vi "生成报告old.vi"() -> ()   [LabVIEW 2013]
uses:
  <vilib>/Utility/NIReport.llb/NI_report.lvclass
  <vilib>/Utility/NIReport.llb/Append Report Text (str wrap).vi
  <vilib>/Utility/NIReport.llb/Append Image to Report (path wrap).vi
  <vilib>/Utility/NIReport.llb/Excel/NI_Excel.lvclass
panel:
  out "bmp路径":path
  out "表格路径":path
  out "报表名称":string
  out "封面路径":path
  out "表格模板路径":path
  out "报表路径":path
  out "filenames":string[](array[string])
  out "print flag":bool
  out "图像个数":i32
  in  "油动机实验报告":T1
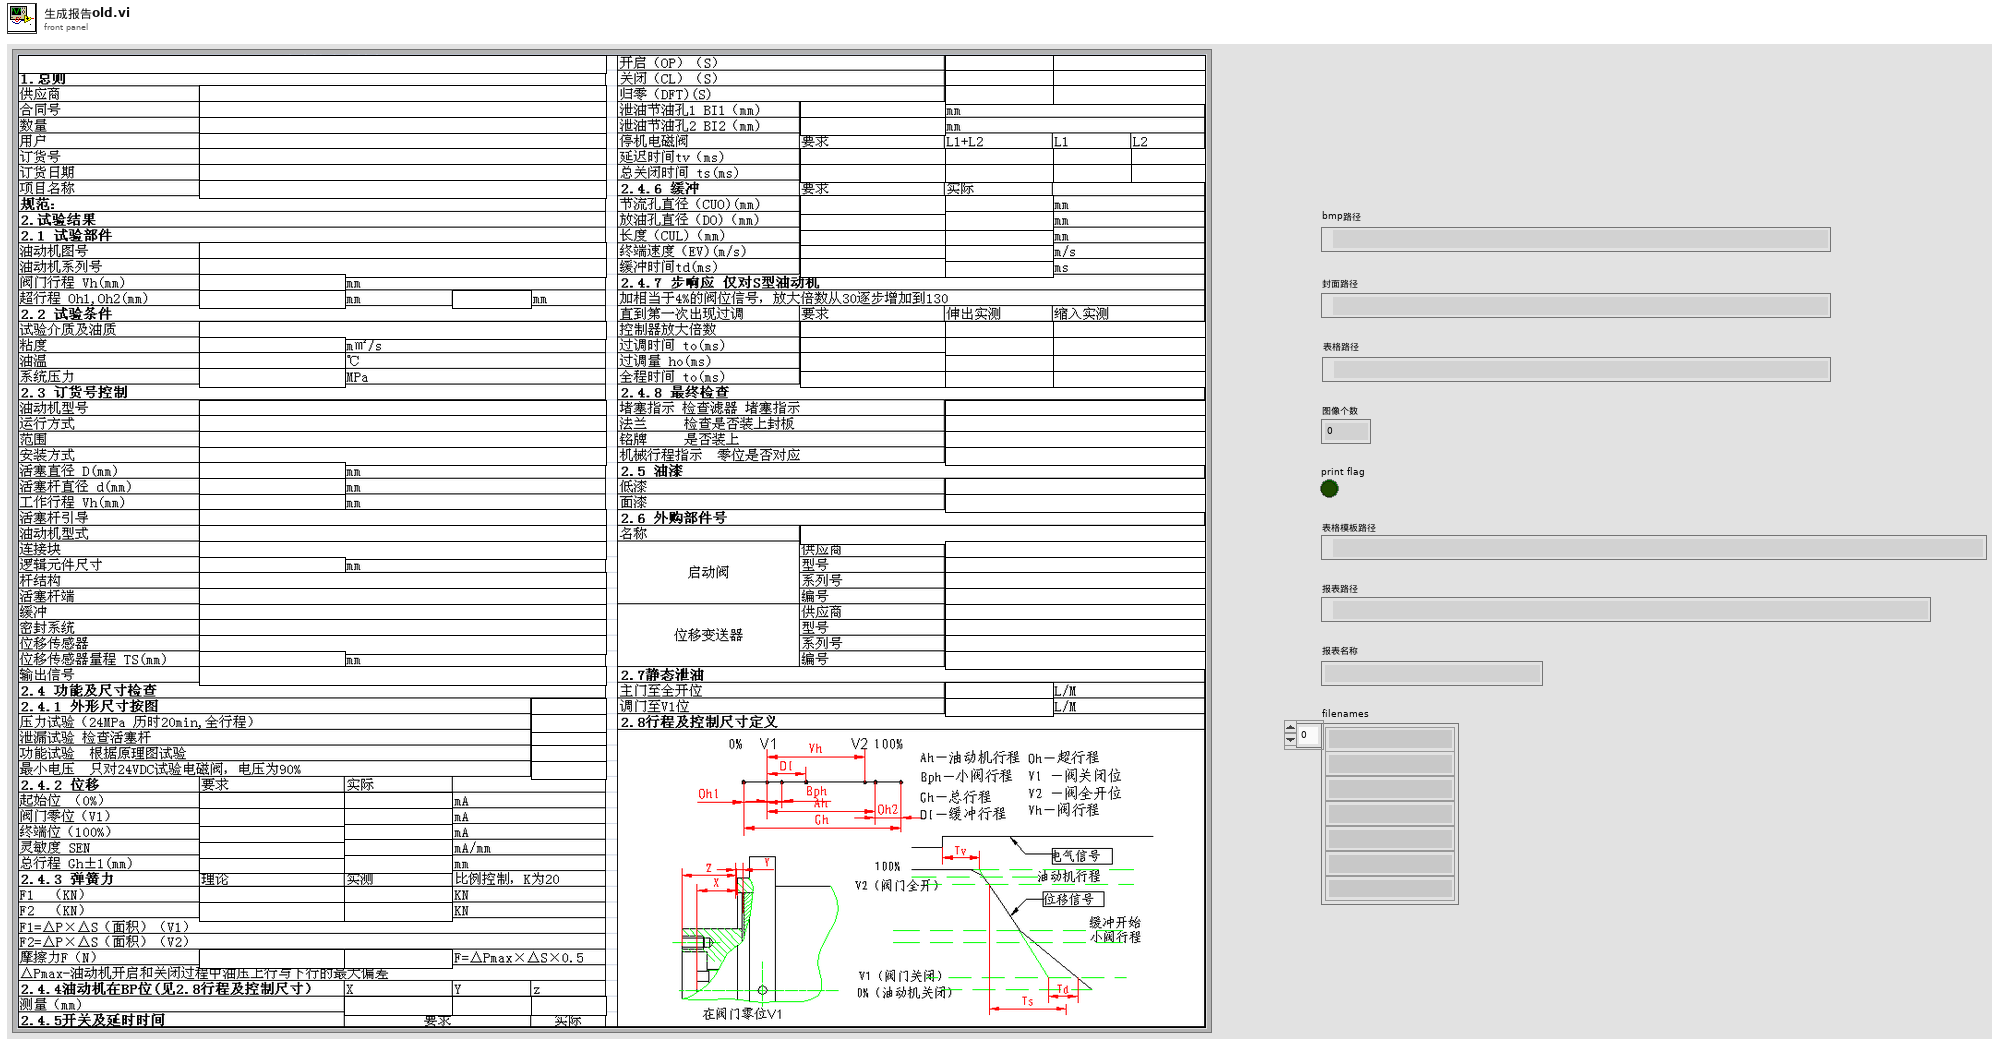
[diagram p1: front panel]
types:
  T1 = cluster{"油动机试验报告名称":string, "供应商1":string, "合同号1":string, "数量1":string, "用户1":string, "订货号1":string, "订货日期1":string, "项目名称1":string, "油动机图号2.1":string, "油动机系列号2.1":string, "阀门行程Vh":string, "试验介质及油质2.2":string, "超行程Oh1":string, "超行程Oh2":string, "粘度2.2":string, "油温2.2":string, "系统压力2.2":string, "油动机型号2.3":string, "运行方式2.3":string, "范围2.3":string, "安装方式2.3":string, "活塞直径D":string, "活塞杆直径d":string, "工作行程Vh2.3":string, "活塞杆引导2.3":string, "油动机型式2.3":string, "连接块2.3":string, "逻辑元件尺寸2.3":string, "杆结构2.3":string, "活塞杆端2.3":string, "缓冲2.3":string, "密封系统2.3":string, "位移传感器2.3":string, "位移传感器量程TS":string, "输出信号":string, "外形尺寸_2.4.1":string, "泄漏试验与否_2.4.1":string, "功能试验与否_2.4.1":string, "最小电压试验与否_2.4.1":string, "压力试验与否_2.4.1":string, "要求起始位2.4.2":string, "实际起始位":string, "要求总行程Gh2.4.2":string, "理论摩擦力F2.4.3":string, "要求灵敏度2.4.2":string, "理论F12.4.3":string, "要求终端位2.4.2":string, "要求阀门零位2.4.2":string, "理论F22.4.3":string, "实际阀门零位V1":string, "实际终端位V2":string, "实际灵敏度SEN":string, "实际总行程Gh":string, "实测F1":string, "实测F2":string, "实测F":string, "油动机在BP位_测量_X":string, "油动机在BP位_测量_Y":string, "油动机在BP位_测量_Z":string, "要求开关延时_开启2.4.5":string, "实际OP":string, "要求开关延时_关闭2.4.5":string, "实际CL":string, "要求开关延时_归零2.4.5":string, "实际DFT":string, "泄油节油孔1_BI1_2.4.5":string, "泄油节油孔2_BI2_2.4.5":string, "要求延迟时间tv_2.4.5":string, "要求总关闭时间ts_2.4.5":string, "要求_终端速度_2.4.6":string, "要求_长度_2.4.6":string, "要求_放油孔直径_2.4.6":string, "要求_节流孔直径_2.4.6":string, "延迟时间L1L2":string, "延迟时间L1":string, "延迟时间L2":string, "总关闭时间L1L2":string, "总关闭时间L1":string, "总关闭时间L2":string, "实际_节流孔直径_2.4.6":string, "缓冲时间td":string, "实际终端速度":string, "实际_长度_2.4.6":string, "实际_放油孔直径_2.4.6":string, "要求_缓冲时间_2.4.6":string, "控制器放大倍数_2.4.7":string, "伸出实测_控制器放大倍数_2.4.7":string, "缩入实测_控制器放大倍数_2.4.7":string, "要求_全程时间_2.4.7":string, "要求_过调时间_2.4.7":string, "要求_过调量_2.4.7":string, "伸出实测_全程时间":string, "伸出实测_过调量":string, "伸出实测_过调时间":string, "缩入实测_全程时间":string, "缩入实测_过调量":string, "缩入实测_过调时间":string, "堵塞指示_2.4.8":string, "法兰_2.4.8 ":string, "铭牌_2.4.8 ":string, "机械行程指示_2.4.8 ":string, "低漆_2.5":string, "面漆_2.5":string, "名称_2.6":string, "启动阀_供应商_2.6":string, "启动阀_型号_2.6":string, "启动阀_系列号_2.6":string, "启动阀_编号_2.6":string, "位移变送器_供应商_2.6":string, "位移变送器_型号_2.6":string, "位移变送器_系列号_2.6":string, "位移变送器_编号_2.6":string, "主门至全开位_2.7":string, "调门至V1位_2.7":string}
  T2 = enum16{"maximized", "minimized", "normal", "no change"}
  T3 = enum16{"Standard Report", "HTML", "Word", "Excel"}
  T4 = cluster{"position (excel)":cluster{"row":i32, "column":i32}, "name (excel)":string, "bookmark (word)":string}
  T5 = cluster{"Italic":enum16{"Italic Unchanged", "Italic On", "Italic Off"}, "Strike Through":enum16{"Strike Through Unchanged", "Strike Through On", "Strike Through Off"}, "Underline":enum16{"Underline Unchanged", "Underline On", "Underline Off"}, "Bold":enum16{"Bold Unchanged", "Bold On", "Bold Off"}}
  T6 = cluster{"Charset (-1)":i16, "Weight (-1)":i16, "Name":string, "Size":string}
  T7 = cluster{"position (excel)":cluster{"row":i32, "column":i32}, string, "bookmark (word)":string}
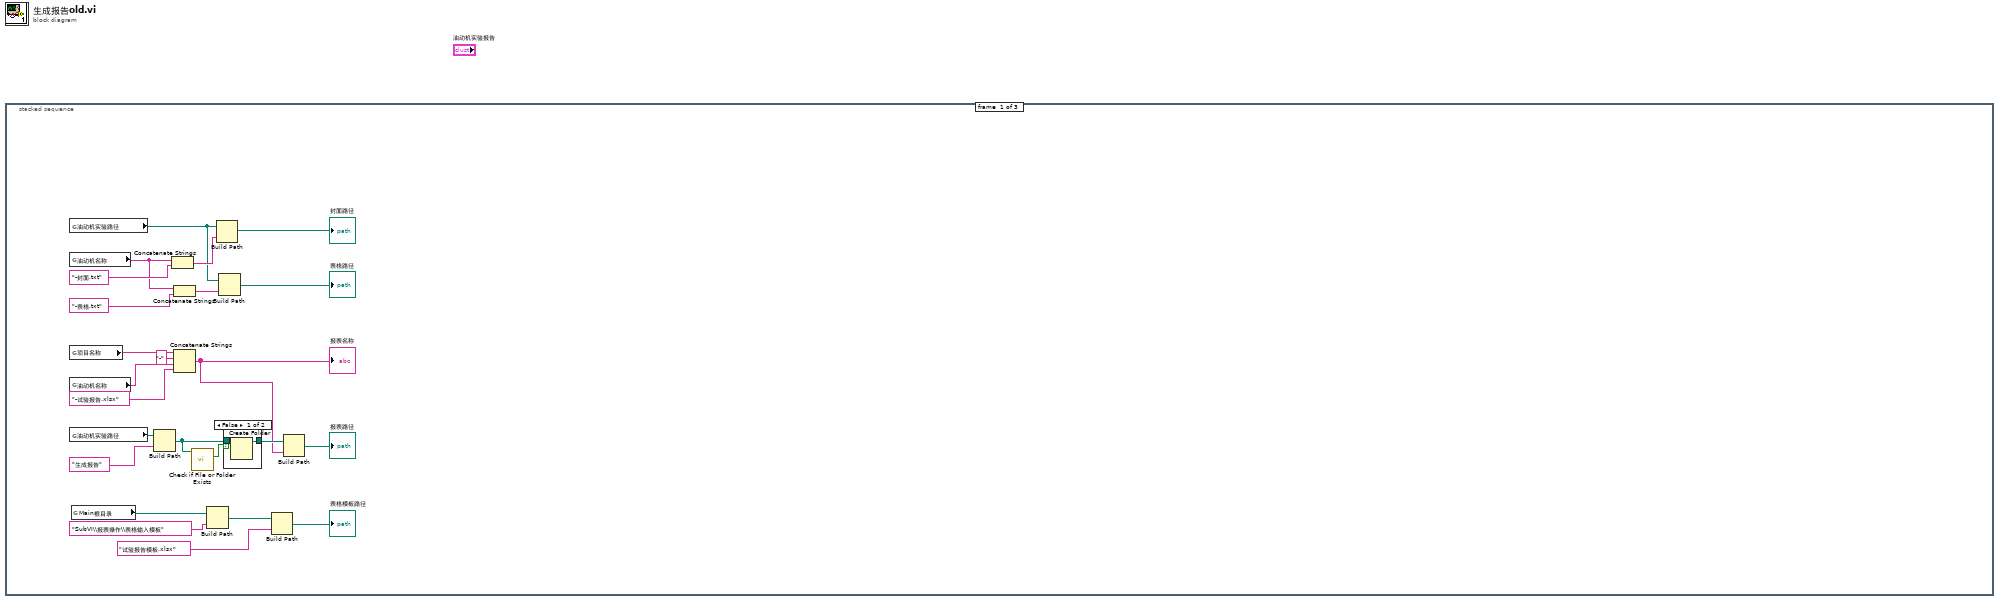
[diagram p0: block diagram]
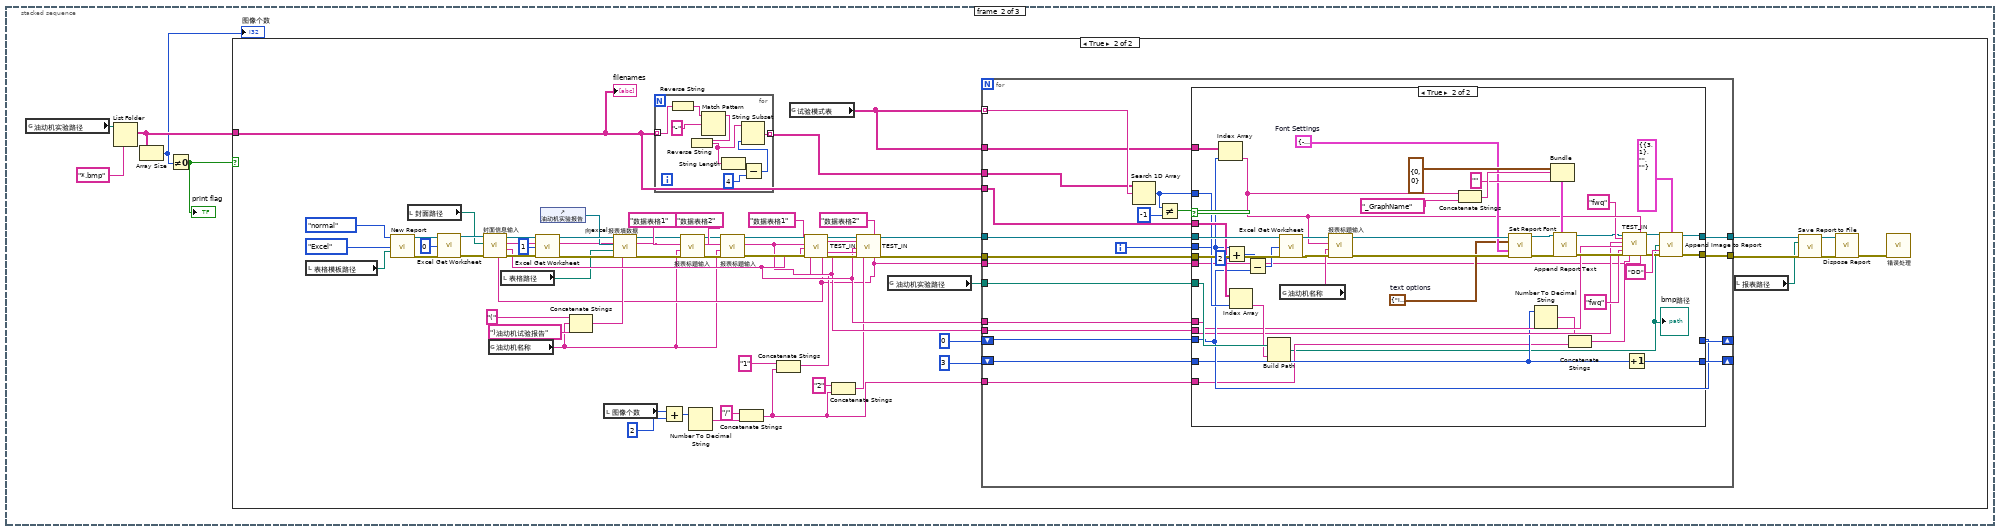
[diagram p3: hidden frame]
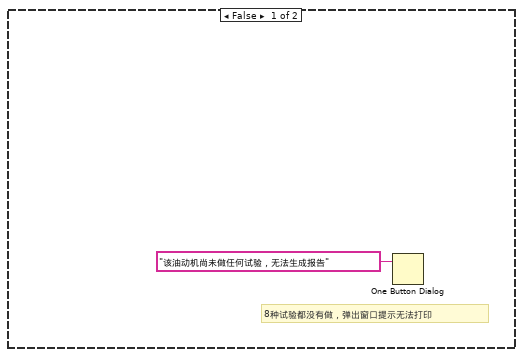
[diagram p4: hidden frame]
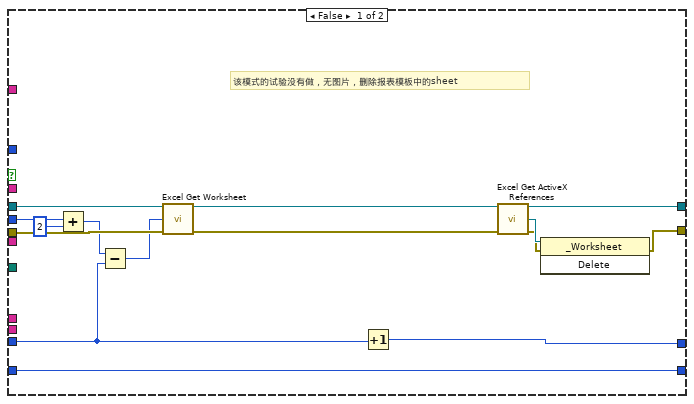
[diagram p5: hidden frame]
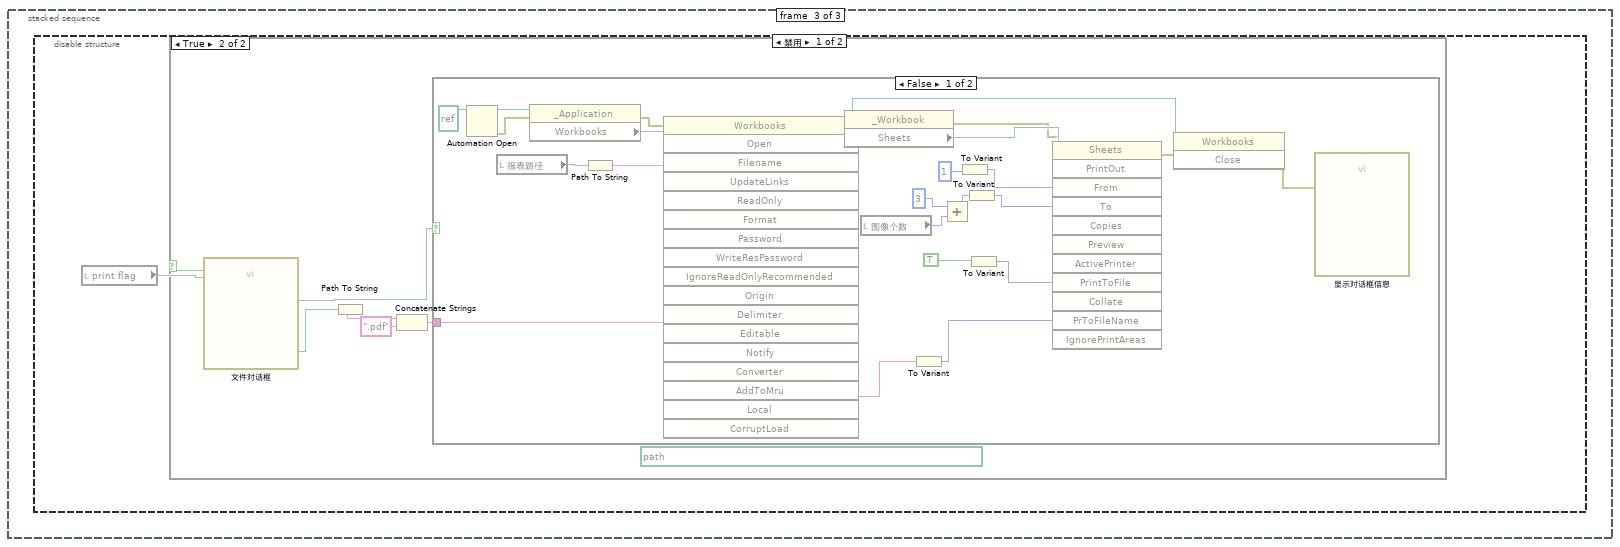
[diagram p6: hidden frame]
diagram:
  n1 = stacked-sequence {
    frame #0 {
      n2 = global read "油动机实验路径.vi" "油动机实验路径"() -> (w8:path)
      n3 = global read "油动机名称.vi" "油动机名称"() -> (w9:string)
      n4 = global read "项目名称.vi" "项目名称"() -> (w20:string)
      n5 = global read "油动机名称.vi" "油动机名称"() -> (w22:string)
      n6 = global read "油动机实验路径.vi" "油动机实验路径"() -> (w14:path)
      n7 = global read "Main根目录.vi" "Main根目录"() -> (w1:path)
      n8 = Build Path(base path=w14, name or relative path="生成报告" ("名称或相对路径")) -> (appended path=w16:path)
      n9 = Concatenate Strings(w9, "-封面.txt" ("名称或相对路径")) -> (w23:string)
      n10 = Concatenate Strings(w9, "-表格.txt" ("名称或相对路径")) -> (w7:string)
      n11 = Concatenate Strings(w20, "-" ("字符串"), w22, "-试验报告.xlsx" ("字符串")) -> (w11:string)
      "报表名称" <- w11
      n12 = call <vilib>:"Check if File or Folder Exists.vi"("path"=w16) -> ("file or folder exists?"=w15:bool)  [unwired: 8 in, 2 out]
      n13 = Build Path(base path=w1, name or relative path="SubVI\\报表操作\\表格输入模板" ("名称或相对路径")) -> (appended path=w2:path)
      n14 = Build Path(base path=w8, name or relative path=w23) -> (appended path=→"封面路径":path)
      n15 = Build Path(base path=w8, name or relative path=w7) -> (appended path=→"表格路径":path)
      n16 = case shown="False" w15 {
        tunnel: [w26 w27] -> w17
        tunnel: w16 -> [w25 w27]
        frame False {
          n17 = Create Folder(path (use dialog)=w25) -> (created path=w26:path)  [unwired: 2 in, 2 out]
        }
        frame True {
        }
      }
      n18 = Build Path(base path=w2, name or relative path="试验报告模板.xlsx" ("名称或相对路径")) -> (appended path=→"表格模板路径":path)
      n19 = Build Path(base path=w17, name or relative path=w11) -> (appended path=→"报表路径":path)
    }
    frame #1 {
      n20 = global read "油动机实验路径.vi" "油动机实验路径"() -> (w28:path)
      n21 = List Folder(path=w28, pattern="*.bmp" ("模式")) -> (filenames=w31:string[])  [unwired: 2 in, 3 out]
      n22 = Array Size(array=w31) -> (size(s)=w30:i32)
      "图像个数" <- w30
      n23 = Not Equal To 0?(x=w30) -> (x != 0?=w29:bool)
      "print flag" <- w29
      n24 = case shown="True" w29 {
        tunnel: w31 -> [_ w77]
        frame False {
          # "8种试验都没有做，弹出窗口提示无法打印"
          n25 = One Button Dialog(message="该油动机尚未做任何试验，无法生成报告" ("消息")) -> ()  [unwired: 1 in, 1 out]
        }
        frame True {
          n26 = local read "表格模板路径"() -> (w39:path)
          n27 = call <vilib>:"New Report.vi"("window state (normal)"=T2."normal", "report type"=T3."Excel", "template (empty)"=w39) -> ("report out"=w72:refnum<class "NI_report.lvclass">, "error out"=w71:errorcluster)  [unwired: 11 in]
          n28 = local read "封面路径"() -> (w42:path)
          n29 = call <vilib>:"Excel Get Worksheet.vi"("report in"=w72, "worksheet index (0)"=0, "error in (no error)"=w71) -> ("report out"=w70:refnum<class "NI_report.lvclass">, "error out"=w69:errorcluster)  [unwired: 11 in]
          n30 = call "封面信息输入.vi"("错误输入（无错误）"=w69, "configuration file path"=w42, "NI_report输入"=w70) -> ("错误输出"=w73:errorcluster, "版本号"=w57:string, "编号"=w56:string, "NI_report输出"=w74:refnum<class "NI_report.lvclass">, "试验日期"=w43:string)  [unwired: 4 in]
          n31 = global read "油动机名称.vi" "油动机名称"() -> (w38:string)
          n32 = local read "表格路径"() -> (w40:path)
          n33 = call <vilib>:"Excel Get Worksheet.vi"("report in"=w74, "worksheet index (0)"=1, "error in (no error)"=w73) -> ("report out"=w86:refnum<class "NI_report.lvclass">, "error out"=w87:errorcluster)  [unwired: 11 in]
          n34 = control-ref of="油动机实验报告"() -> (w85:refnum<vi>)
          n35 = Concatenate Strings("(" ("字符串"), w38, ")油动机试验报告" ("字符串")) -> (w44:string)
          n36 = local read "图像个数"() -> (w55:i32)
          n37 = call "向excel报表填数据.vi"("报告抬头"=w44, "错误输入（无错误）"=w87, "报表路径"=w40, "Cluster引用句柄"=w85, "NI_report输入"=w86) -> ("错误输出"=w88:errorcluster, "NI_report输出"=w89:refnum<class "NI_report.lvclass">)  [unwired: 5 in]
          n38 = for {
            tunnel: w77 -> [w100] mode=indexing
            tunnel: [w103] -> w78 mode=indexing
            n39 = Reverse String(1:w100) -> (0:w101:string)
            n40 = Match Pattern(string=w101, regular expression="-" ("正则表达式")) -> (before substring=w99:string)  [unwired: 1 in, 3 out]
            n41 = Reverse String(1:w99) -> (0:w95:string)
            n42 = String Length(string=w95) -> (length=w98:i32)
            n43 = Subtract(x=w98, y=4) -> (x-y=w96:i32)
            n44 = String Subset(string=w95, length (rest)=w96) -> (substring=w103:string)  [unwired: 1 in]
          }
          n45 = Add(x=w55, y=2) -> (x+y=w53:i32)
          n46 = call "报表标题输入.vi"("错误输入（无错误）"=w88, "油动机名称"=w38, "_sheet_name"="数据表格1", "NI_report输入"=w89) -> ("错误输出"=w91:errorcluster, "NI_report输出"=w92:refnum<class "NI_report.lvclass">)  [unwired: 6 in]
          n47 = Number To Decimal String(number=w53) -> (decimal integer string=w52:string)  [unwired: 1 in]
          n48 = call "报表标题输入.vi"("错误输入（无错误）"=w91, "油动机名称"=w38, "_sheet_name"="数据表格2", "NI_report输入"=w92) -> ("错误输出"=w60:errorcluster, "NI_report输出"=w59:refnum<class "NI_report.lvclass">)  [unwired: 6 in]
          n49 = Concatenate Strings("/" ("字符串"), w52) -> (w35:string)
          n50 = Concatenate Strings("1" ("页码"), w35) -> (w47:string)
          n51 = global read "试验模式表.vi" "试验模式表"() -> (w36:string[])
          n52 = call "TEST_IN.vi"("NI_report输入"=w59, "编号"=w56, "版本"=w57, "错误输入（无错误）"=w60, "页码"=w47, "_sheet_name"="数据表格1", "试验日期"=w43) -> ("NI_report输出"=w67:refnum<class "NI_report.lvclass">, "试验员out"=w64:string, "检查员out"=w65:string, "错误输出"=w66:errorcluster)  [unwired: 9 in]
          n53 = Concatenate Strings("2" ("页码"), w35) -> (w48:string)
          n54 = call "TEST_IN.vi"("NI_report输入"=w67, "试验员"=w64, "编号"=w56, "版本"=w57, "检查员"=w65, "错误输入（无错误）"=w66, "页码"=w48, "_sheet_name"="数据表格2", "试验日期"=w43) -> ("NI_report输出"=w62:refnum<class "NI_report.lvclass">, "错误输出"=w61:errorcluster)  [unwired: 7 in, 2 out]
          n55 = global read "油动机实验路径.vi" "油动机实验路径"() -> (w37:path)
          n56 = for {
            tunnel: w36 -> [w124] mode=indexing
            tunnel: w77 -> [w114]
            tunnel: w37 -> [w116]
            tunnel: w36 -> [w113]
            shift-right: [w111] -> _
            shift-left: 0 -> [w112]
            shift-right: [w109] -> _
            shift-left: 3 -> [w110]
            tunnel: w78 -> [w108]
            tunnel: w62 -> [w118]
            tunnel: [w120] -> w80
            tunnel: w61 -> [w117]
            tunnel: [w119] -> w79
            tunnel: w57 -> [w107]
            tunnel: w56 -> [w106]
            tunnel: w35 -> [w105]
            tunnel: w43 -> [w104]
            i -> [w121]
            n57 = Search 1D Array(1D array=w108, element=w124) -> (index of element=w115:i32)  [unwired: 1 in]
            n58 = Not Equal?(x=w115, y=-1) -> (x != y?=w122:bool)
            n59 = case shown="True" w122 {
              tunnel: w121 -> [w130 w167]
              tunnel: [w135 w182] -> w120
              tunnel: [w134 w179] -> w119
              tunnel: w118 -> [w133 w181]
              tunnel: w117 -> [w132 w180]
              tunnel: w116 -> [_ w176]
              tunnel: w115 -> [_ w177]
              tunnel: w114 -> [_ w178]
              tunnel: w113 -> [_ w173]
              tunnel: w112 -> [w127 w168]
              tunnel: [w131 w168] -> w111
              tunnel: w110 -> [w125 w145]
              tunnel: [w125 w172] -> w109
              tunnel: w107 -> [_ w147]
              tunnel: w106 -> [_ w146]
              tunnel: w105 -> [_ w144]
              tunnel: w104 -> [_ w141]
              frame False {
                # "该模式的试验没有做，无图片，删除报表模板中的sheet"
                n60 = Add(x=w130, y=2) -> (x+y=w128:i32)
                n61 = Subtract(x=w128, y=w127) -> (x-y=w126:i32)
                n62 = call <vilib>:"Excel Get Worksheet.vi"("report in"=w133, "worksheet index (0)"=w126, "error in (no error)"=w132) -> ("report out"=w137:refnum<class "NI_report.lvclass">, "error out"=w136:errorcluster)  [unwired: 11 in]
                n63 = Increment(x=w127) -> (x+1=w131:i32)
                n64 = call <vilib>:"Excel Get ActiveX References.vi"("report in"=w137, "error in (no error)"=w136) -> ("report out"=w135:refnum<class "NI_report.lvclass">, "Excel._Worksheet"=w139:refnum<k7>, "error out"=w138:errorcluster)  [unwired: 7 in, 4 out]
                n65 = invoke class="_Worksheet" method="Delete"(reference=w139, error in=w138) -> (error out=w134:errorcluster)  [unwired: 1 in, 2 out]
              }
              frame True {
                w155 = T5 {"Italic"=enum."Italic Unchanged", "Strike Through"=enum."Strike Through Unchanged", "Underline"=enum."Underline Unchanged", "Bold"=enum."Bold On"}  # text options
                w156 = T6 {"Charset (-1)"=-1, "Weight (-1)"=-1, "Name"="宋体", "Size"="12"}  # Font Settings
                n66 = Index Array(array=w173, index=w167) -> (element=w154:string)
                n67 = Add(x=w167, y=2) -> (x+y=w169:i32)
                n68 = Index Array(array=w178, index=w177) -> (element=w175:string)
                n69 = Subtract(x=w169, y=w168) -> (x-y=w166:i32)
                n70 = Build Path(base path=w176, name or relative path=w175) -> (appended path=w140:path)
                "bmp路径" <- w140
                n71 = call <vilib>:"Excel Get Worksheet.vi"("report in"=w181, "worksheet index (0)"=w166, "error in (no error)"=w180) -> ("report out"=w184:refnum<class "NI_report.lvclass">, "error out"=w185:errorcluster)  [unwired: 11 in]
                n72 = global read "油动机名称.vi" "油动机名称"() -> (w174:string)
                n73 = call "报表标题输入.vi"("错误输入（无错误）"=w185, "油动机名称"=w174, "_sheet_name"=w154, "NI_report输入"=w184) -> ("错误输出"=w159:errorcluster, "NI_report输出"=w160:refnum<class "NI_report.lvclass">)  [unwired: 6 in]
                n74 = Concatenate Strings(w154, "_GraphName" ("字符串")) -> (w164:string)
                n75 = call-dynamic "Set Report Font.vi"("report in"=w160, "text options"=w155, "font settings"=w156, "error in (no error)"=w159) -> ("report out"=w158:refnum<class "NI_report.lvclass">, "error out"=w157:errorcluster)  [unwired: 9 in, 1 out]
                n76 = Number To Decimal String(number=w145) -> (decimal integer string=w143:string)  [unwired: 1 in]
                n77 = Bundle("position (excel)"=cluster{"row":i32, "column":i32} {"row"=0, "column"=0}, w164, "bookmark (word)"="") -> (w165:T7)  [unwired: 1 in]
                n78 = call-poly <vilib>:"Append Report Text.vi"("report in"=w158, "MS Office parameters"=w165, "error in (no error)"=w157) -> ("report out"=w152:refnum<class "NI_report.lvclass">, "error out"=w149:errorcluster)  [unwired: 9 in, 2 out]
                n79 = Concatenate Strings(w143, w144) -> (w142:string)
                n80 = call "TEST_IN.vi"("NI_report输入"=w152, "试验员"="fwq", "编号"=w146, "版本"=w147, "检查员"="fwq" ("试验员"), "错误输入（无错误）"=w149, "页码"=w142, "_sheet_name"=w154, "试验日期"=w141) -> ("NI_report输出"=w151:refnum<class "NI_report.lvclass">, "错误输出"=w150:errorcluster)  [unwired: 7 in, 2 out]
                n81 = Increment(x=w145) -> (x+1=w172:i32)
                n82 = call-poly <vilib>:"Append Image to Report.vi"("report in"=w151, "MS Office parameters"=T4 {"position (excel)"={"row"=3, "column"=1}, "name (excel)"="", "bookmark (word)"=""}, "path or URL of image"=w140, "caption or alternative string"="DD", "error in (no error)"=w150) -> ("report out"=w182:refnum<class "NI_report.lvclass">, "error out"=w179:errorcluster)  [unwired: 7 in, 2 out]
              }
            }
          }
          n83 = local read "报表路径"() -> (w41:path)
          n84 = call-dynamic "Save Report to File.vi"("report in"=w80, "report file path"=w41, "error in (no error)"=w79) -> ("report out"=w76:refnum<class "NI_report.lvclass">, "error out"=w75:errorcluster)  [unwired: 11 in]
          n85 = call-dynamic "Dispose Report.vi"("report in"=w76, "error in (no error)"=w75) -> ("error out"=w34:errorcluster)  [unwired: 13 in]
          n86 = call "错误处理.vi"("error in (no error)"=w34) -> ()  [unwired: 2 in]
          "filenames" <- w77
        }
      }
    }
    frame #2 {
      n87 = disable-structure shown="禁用" {
        frame Disabled {
          n88 = local read "print flag"() -> (w186:bool)
          n89 = case shown="True" w186 {
            frame False {
            }
            frame True {
              (unwired) path "C:/Documents and Settings/Administrator/桌面/new3.pdf" ("file path")
              n90 = call "文件对话框"() -> ("selected path"=w189:path, "cancelled"=w188:bool)  [unwired: 12 in, 2 out]
              n91 = Path To String(path=w189) -> (string=w190:string)
              n92 = Concatenate Strings(w190, ".pdf" ("字符串")) -> (w187:string)
              n93 = case shown="False" w188 {
                tunnel: w187 -> [w192 _]
                frame False {
                  n94 = Automation Open(Automation Refnum=refnum<k7> refnum ("Excel._Application")) -> (Automation Refnum=w214:refnum<k7>, error out=w207:errorcluster)  [unwired: 3 in]
                  n95 = local read "报表路径"() -> (w203:path)
                  n96 = property class="_Application"(reference=w214, error in=w207) -> (error out=w208:errorcluster, "Workbooks"=w213:refnum<k7>)  [unwired: 1 out]
                  n97 = Path To String(path=w203) -> (string=w196:string)
                  n98 = invoke class="Workbooks" method="Open"(reference=w213, error in=w208, "Filename"=w196) -> (reference out=w199:refnum<k7>, error out=w209:errorcluster, "Open"=w212:refnum<k7>)  [unwired: 15 in, 15 out]
                  n99 = property class="_Workbook"(reference=w212, error in=w209) -> (error out=w210:errorcluster, "Sheets"=w211:refnum<k7>)  [unwired: 1 out]
                  n100 = local read "图像个数"() -> (w201:i32)
                  n101 = To Variant(anything=w192) -> (Variant=w193:variant)
                  n102 = Add(x=3, y=w201) -> (x+y=w200:i32)
                  n103 = To Variant(anything=1) -> (Variant=w205:variant)
                  n104 = To Variant(anything=w200) -> (Variant=w204:variant)
                  n105 = To Variant(anything=TRUE) -> (Variant=w194:variant)
                  n106 = invoke class="Sheets" method="PrintOut"(reference=w211, error in=w210, "From"=w205, "To"=w204, "PrintToFile"=w194, "PrToFileName"=w193) -> (error out=w198:errorcluster)  [unwired: 6 in, 11 out]
                  n107 = invoke class="Workbooks" method="Close"(reference=w199, error in=w198) -> (error out=w197:errorcluster)  [unwired: 1 in, 2 out]
                  n108 = call "显示对话框信息"("error in (no error)"=w197) -> ()  [unwired: 9 in, 2 out]
                }
                frame True {
                }
              }
            }
          }
        }
        frame Enabled {
        }
      }
    }
  }
